vi "central pos and width (SubVI).vi"(2 "threshold level [0-1]":dbl=0.2 format="%#_13g", 3 "proj profile":dbl[](array[numeric])) -> (0 "width":dbl, 1 "center pos":dbl)   [LabVIEW 2024]
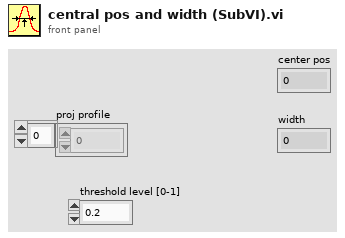
[diagram p1: front panel]
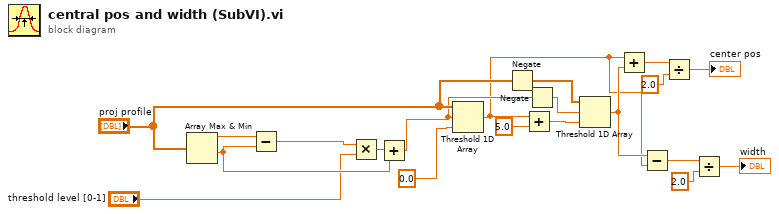
[diagram p0: block diagram]
diagram:
  n1 = Array Max & Min(array="proj profile") -> (max value=w14:dbl, min value=w16:dbl)  [unwired: 2 out]
  n2 = Subtract(x=w14, y=w16) -> (x-y=w15:dbl)
  n3 = Multiply(x=w15, y="threshold level [0-1]") -> (x*y=w17:dbl)
  n4 = Add(x=w17, y=w16) -> (x+y=w18:dbl)
  n5 = Threshold 1D Array(1:0.0, 2:w18, 3:"proj profile") -> (0:w5:dbl)
  n6 = Negate(x="proj profile") -> (-x=w12:dbl[])
  n7 = Add(x=w5, y=5.0) -> (x+y=w8:dbl)
  n8 = Negate(x=w18) -> (-x=w11:dbl)
  n9 = Threshold 1D Array(1:w8, 2:w11, 3:w12) -> (0:w6:dbl)
  n10 = Add(x=w5, y=w6) -> (x+y=w10:dbl)
  n11 = Subtract(x=w6, y=w5) -> (x-y=w3:dbl)
  n12 = Divide(x=w10, y=2.0) -> (x/y=→"center pos":dbl)
  n13 = Divide(x=w3, y=2.0) -> (x/y=→"width":dbl)
